vi "SetHome2.vi"(8 "error in (no error)":errorcluster, 10 "N Ax":dbl, 11 "CU ID":i32) -> (0 "error out":errorcluster)   [LabVIEW 2021]
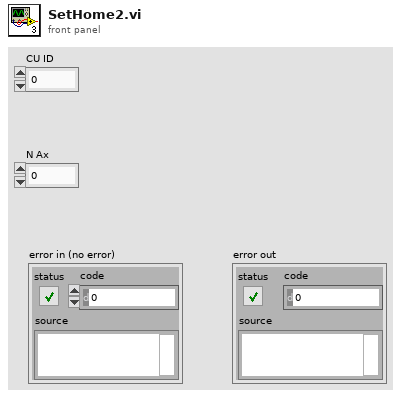
[diagram p1: front panel]
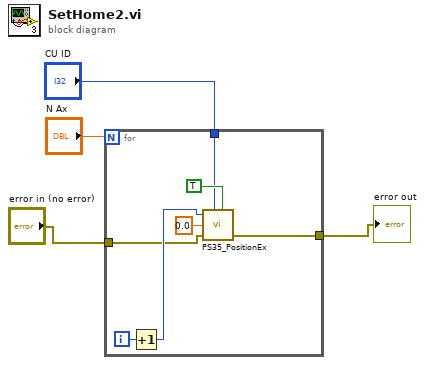
[diagram p0: block diagram]
diagram:
  n1 = for {
    N: "N Ax" -> [_]
    tunnel: "CU ID" -> [w7]
    tunnel: [w6] -> w1
    tunnel: "error in (no error)" -> [w5]
    i -> [w9]
    n2 = Increment(x=w9) -> (x+1=w8:i32)
    n3 = call "PS35_PositionEx.vi"("Axis number"=w8, "Control unit ID"=w7, "dValue-In"=0.0, "error in (no error)"=w5, "function"=TRUE) -> ("error out"=w6:errorcluster)  [unwired: 3 in, 1 out]
  }
  "error out" <- w1
